vi "PulsehistogramSimple_NI5771.vi"() -> ()   [LabVIEW 2012]
uses:
  <vilib>/Platform/TimedLoop/XDataNode/timing_clust.ctl
  <vilib>/Platform/TimedLoop/XDataNode/nitl_modes.ctl
  <vilib>/Platform/TimedLoop/XDataNode/wakeup.ctl
  <vilib>/rvi/eio/common/nirviEmuTemplateMethod_errors.vi
  <vilib>/rvi/Emulation/niFpgaSctlEmulationRegisterWithScheduler.vi
  <vilib>/rvi/interface/RandomDataEmulation/nirviRandomDataFPGAFIFO.vi
  <vilib>/rvi/interface/RandomDataEmulation/niFpgaRandomDataHandleErrors.vi
  <vilib>/rvi/Emulation/niFpgaSctlEmulationScheduler.vi
  <vilib>/Platform/TimedLoop/XDataNode/XDataNode.xnode
  <vilib>/eio/EIONode/EIONode.xnode
  <vilib>/rvi/DataTransferAndStorage/Container/XNode/niFpgaContainer.xnode
  <vilib>/rvi/interface/RandomDataEmulation/nirviRandomDataFpgaReadWriteTemplate.vi
  <vilib>/Platform/TimedLoop/XDataNode/XDNodeRunTimeDep.lvlib
panel:
  out "User Error":bool
  out "ToHostU8FIFO Overflow":bool
  out "ToHostU64FIFO Overflow":bool
  out "IO Module\\AI Over Range":bool
  in  "User Command Commit":bool
  in  "User Command":u8
  out "User Command Idle":bool
  out "User Command Status":u8
  in  "User Data 0":u16
  in  "User Data 1":u8
  out "PLL Locked":bool
  out "User Error":bool
  out "Configured?":bool
  # "Analog acquisition 1.5GHz\nChannel 0 & trigger"
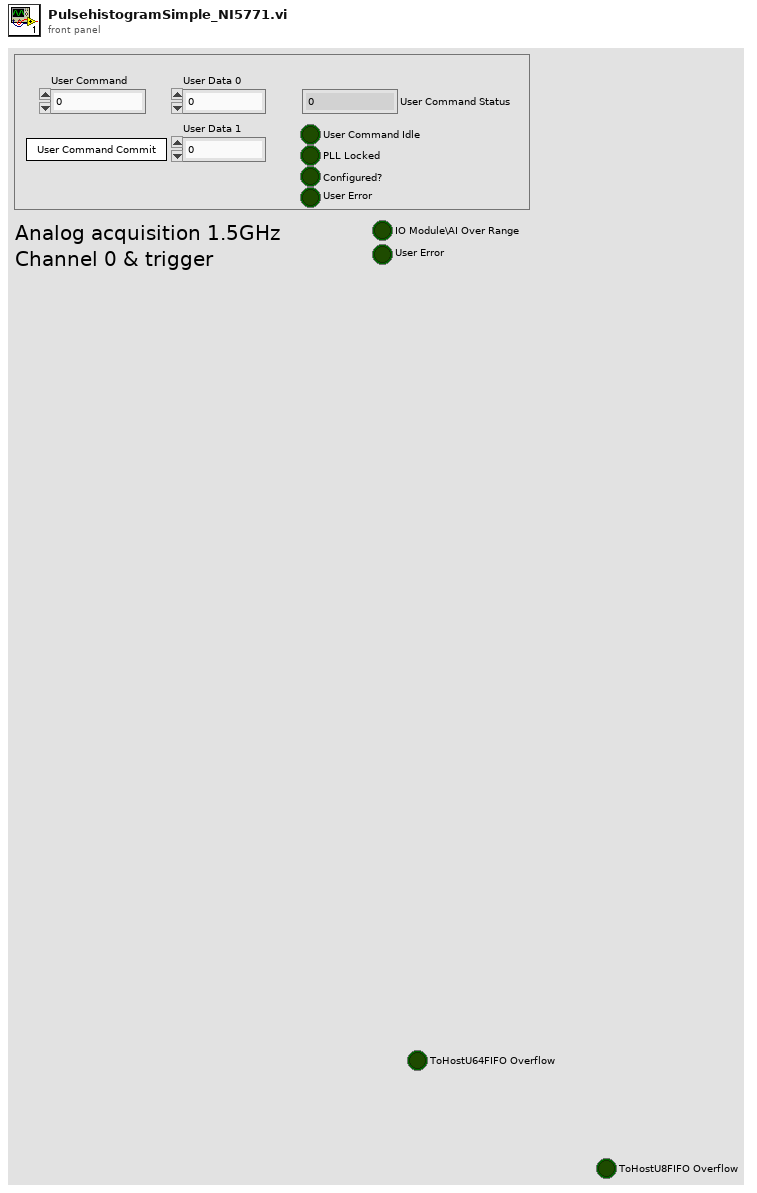
[diagram p1: front panel]
types:
  T1 = typedef "XDNodeRunTimeDep.lvlib/timing_clust.ctl" = cluster{"Expected End [f-1]":u64, "Actual End [f-1]":u64, "Finished Late? [f-1]":bool, "Expected End [i-1]":u64, "Actual End [i-1]":u64, "Finished Late? [i-1]":bool, "Expected Start [i]":u64, "Actual Start [i]":u64, "Expected Start [f]":u64, "Actual Start [f]":u64, "Source Name":string, "Structure Name":string, "Period":i64, "Deadline":i64, "Offset":i64, "Start":i64, "Priority":i32, "Timeout":i32, "Mode":T2, "Wakeup Reason":T3, "Error":errorcluster, "Source Type":string, "Secondary Source Type":string, "Global End Time":u64, "Global Start Time":u64, "Frame Duration":u64, "Iteration Duration":u64, "Assigned CPU":i32, "I/O Scan Engine Mode":u32}
  T2 = typedef "XDNodeRunTimeDep.lvlib/nitl_modes.ctl" = enum32{"No Change", "Process missed periods, maintain original phase", "Discard missed periods, maintain original phase", "Process missed periods, ignore original phase", "Discard missed periods, ignore original phase"}
  T3 = typedef "XDNodeRunTimeDep.lvlib/wakeup.ctl" = enum32{"Normal", "Aborted", "Asynchronous wakeup", "Timing source error", "Timed loop error", "Timeout"}
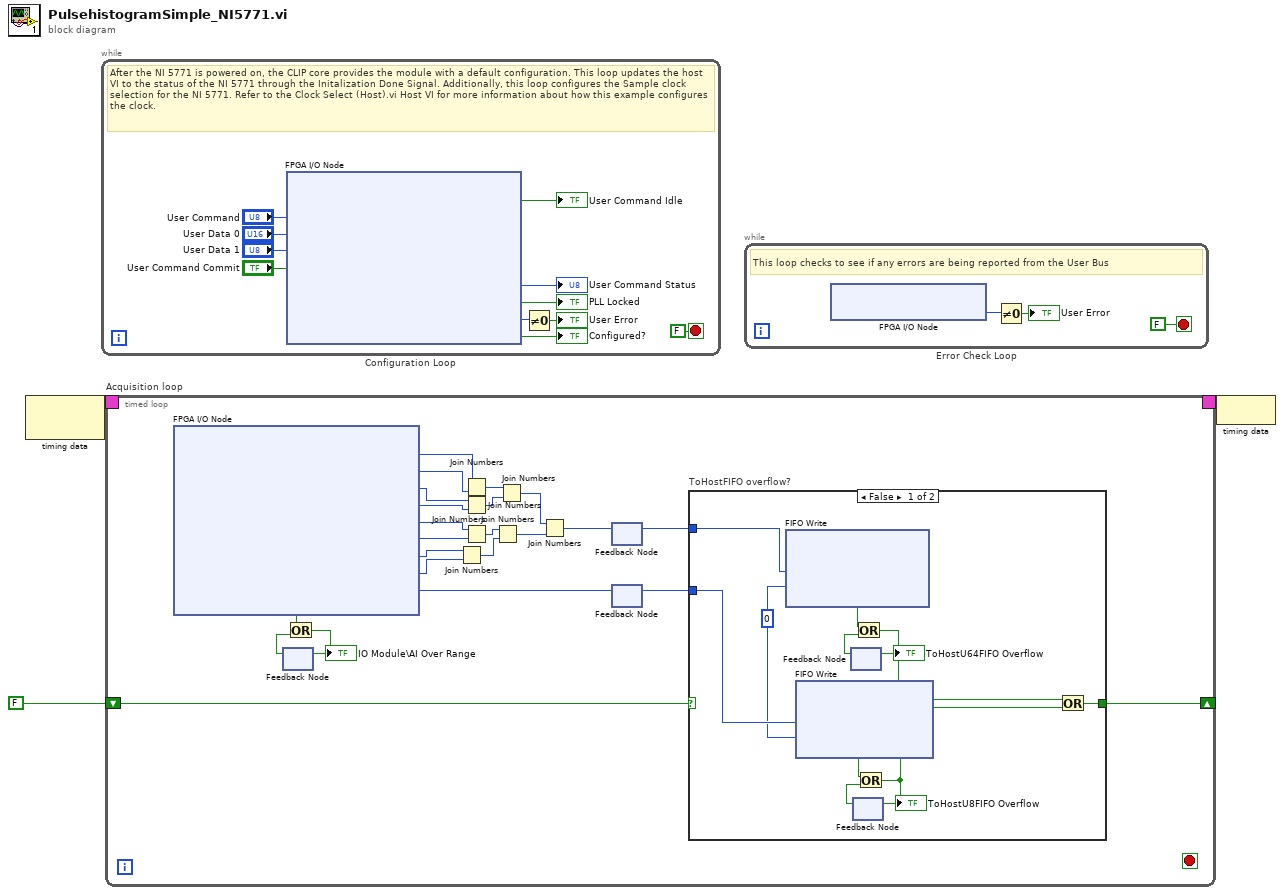
[diagram p0: block diagram]
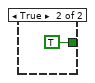
[diagram p2: hidden frame]
diagram:
  n1 = node-c288() -> (w3:T1)  [unwired: 1 in]
  n2 = while "Configuration Loop" {
    stop <- FALSE stop-if-true
    # "After the NI 5771 is powered on, the CLIP core provides the module with a default configuration. This loop updates the host VI to the status of the NI 5771 through the Initalization Done Signal. Additionally, this loop configures the Sample clock selection for the NI 5771. Refer to the Clock Select (Host).vi Host VI for more information about how this example configures the clock."
    n3 = xnode "FPGA I/O Node"("IO Module\\User Command"="User Command", "IO Module\\User Data 0"="User Data 0", "IO Module\\User Data 1"="User Data 1", "IO Module\\User Command Commit"="User Command Commit") -> ("IO Module\\User Command Idle"=→"User Command Idle":bool, "IO Module\\User Command Status"=→"User Command Status":u8, "IO Module\\PLL Locked"=→"PLL Locked":bool, "IO Module\\User Error"=w7:u8, "IO Module\\Initialization Done"=→"Configured?":bool)  [unwired: 9 in, 9 out]
    n4 = Not Equal To 0?(x=w7) -> (x != 0?=→"User Error":bool)
  }
  n5 = timed-loop "Acquisition loop" {
    timing: w3 -> [_]
    timing-out: [_] -> w2
    shift-right: [w20] -> _
    shift-left: FALSE -> [w19]
    stop <- _ stop-if-true
    n6 = xnode "FPGA I/O Node"() -> ("IO Module\\AI 0 Data N-7"=w27:u8, "IO Module\\AI 0 Data N-6"=w28:u8, "IO Module\\AI 0 Data N-5"=w29:u8, "IO Module\\AI 0 Data N-4"=w30:u8, "IO Module\\AI 0 Data N-3"=w31:u8, "IO Module\\AI 0 Data N-2"=w32:u8, "IO Module\\AI 0 Data N-1"=w33:u8, "IO Module\\AI 0 Data N"=w34:u8, "IO Module\\Synchronous Trigger Input"=w16:u8, "IO Module\\AI Over Range"=w37:bool)  [unwired: 10 in, 10 out]
    n7 = feedback #1() -> (w36:bool)  [unwired: 1 in]
    n8 = Or(x=w37, y=w36) -> (x .or. y?=w35:bool)
    "IO Module\\AI Over Range" <- w35
    n9 = feedback-in #1(w35) -> ()
    n10 = Join Numbers(hi=w33, lo=w34) -> ((hi.lo)=w23:u16)
    n11 = Join Numbers(hi=w27, lo=w28) -> ((hi.lo)=w26:u16)
    n12 = Join Numbers(hi=w29, lo=w30) -> ((hi.lo)=w25:u16)
    n13 = Join Numbers(hi=w31, lo=w32) -> ((hi.lo)=w24:u16)
    n14 = Join Numbers(hi=w24, lo=w23) -> ((hi.lo)=w21:u32)
    n15 = Join Numbers(hi=w26, lo=w25) -> ((hi.lo)=w22:u32)
    n16 = Join Numbers(hi=w22, lo=w21) -> ((hi.lo)=w18:u64)
    n17 = feedback-in #2(w18) -> ()
    n18 = feedback #2() -> (w17:u64)  [unwired: 1 in]
    n19 = feedback #3() -> (w15:u8)  [unwired: 1 in]
    n20 = feedback-in #3(w16) -> ()
    n21 = case "ToHostFIFO overflow?" shown="False" w19 {
      tunnel: w17 -> [w47 _]
      tunnel: w15 -> [w44 _]
      tunnel: [w39 TRUE] -> w20
      frame False {
        w38 = 0 ("Timeout")
        n22 = xnode ("FIFO Write")("Element"=w47, "Timeout"=w38) -> ("Timed Out?"=w45:bool)  [unwired: 1 in, 1 out]
        n23 = xnode ("FIFO Write")("Element"=w44, "Timeout"=w38) -> ("Timed Out?"=w42:bool)  [unwired: 1 in, 1 out]
        n24 = feedback #4() -> (w46:bool)  [unwired: 1 in]
        n25 = feedback #5() -> (w43:bool)  [unwired: 1 in]
        n26 = Or(x=w45, y=w46) -> (x .or. y?=w41:bool)
        "ToHostU64FIFO Overflow" <- w41
        n27 = feedback-in #4(w41) -> ()
        n28 = Or(x=w42, y=w43) -> (x .or. y?=w40:bool)
        "ToHostU8FIFO Overflow" <- w40
        n29 = feedback-in #5(w40) -> ()
        n30 = Or(x=w41, y=w40) -> (x .or. y?=w39:bool)
      }
      frame True {
      }
    }
  }
  n31 = while "Error Check Loop" {
    stop <- FALSE stop-if-true
    # "This loop checks to see if any errors are being reported from the User Bus"
    n32 = xnode "FPGA I/O Node"() -> ("IO Module\\User Error"=w52:u8)  [unwired: 1 in, 1 out]
    n33 = Not Equal To 0?(x=w52) -> (x != 0?=→"User Error":bool)
  }
  n34 = node-c288(w2) -> ()
